vi "ReversedEngineering GetStateMachineCaseSelectorRefInfo.vi"(0 "Diagram":refnum<vi>, 1 "WhileLoop(False)":bool, 5 "error in (no error)":errorcluster) -> (12 "OutSideWhileLoopDiagram":refnum<vi>, 14 "StateWhileLoopDiagram":refnum<vi>, 15 "StateMachineCaseSelector":refnum<vi>, 16 "Found":bool, 19 "error out":errorcluster)   [LabVIEW 2016]
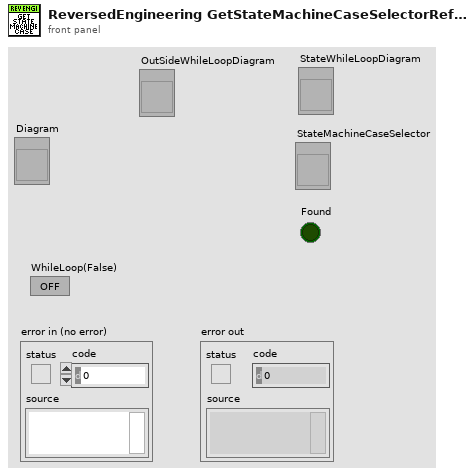
[diagram p1: front panel]
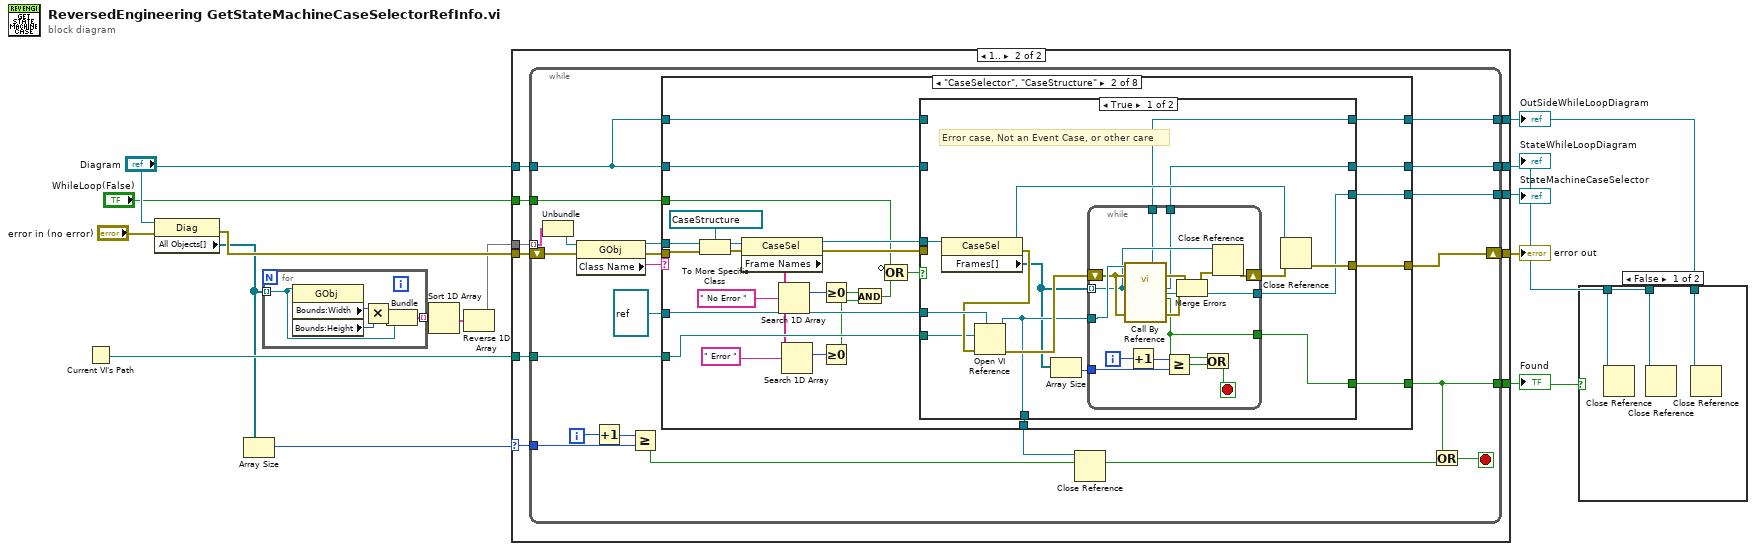
[diagram p0: block diagram]
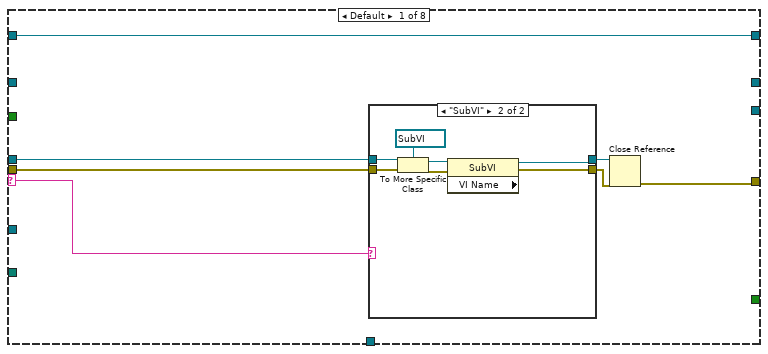
[diagram p3: hidden frame]
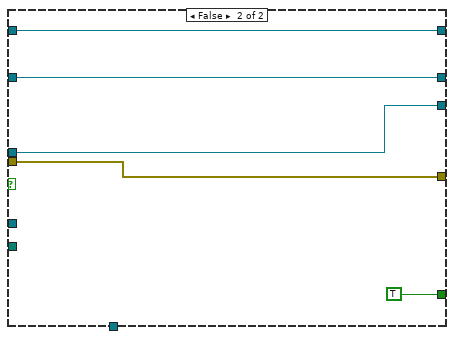
[diagram p5: hidden frame]
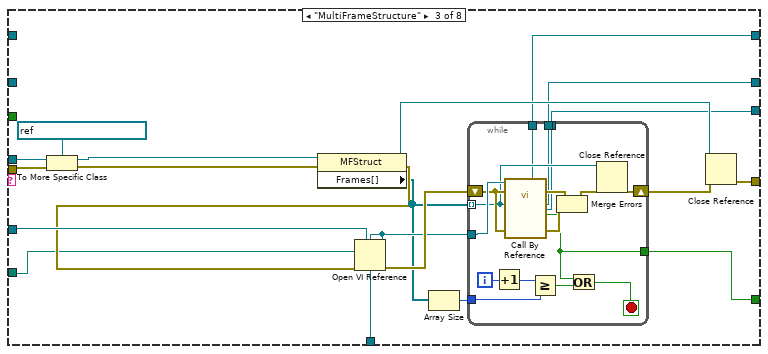
[diagram p6: hidden frame]
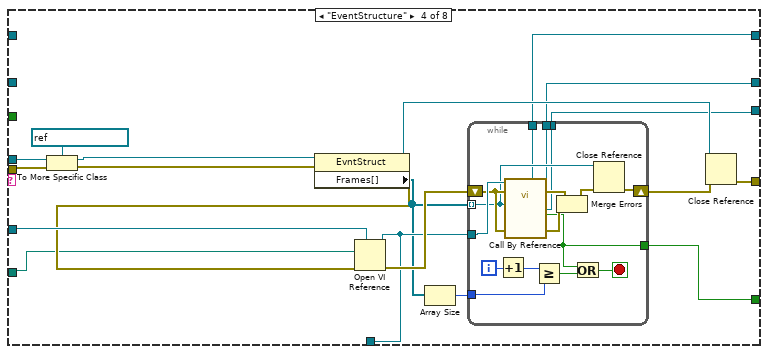
[diagram p7: hidden frame]
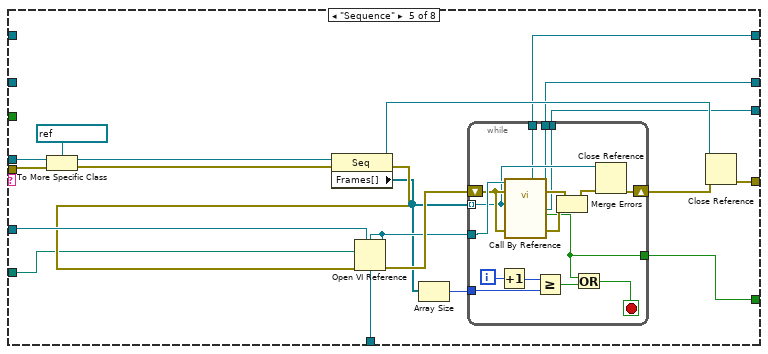
[diagram p8: hidden frame]
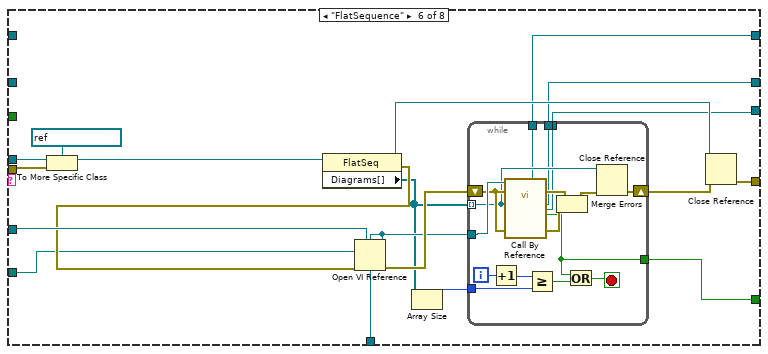
[diagram p9: hidden frame]
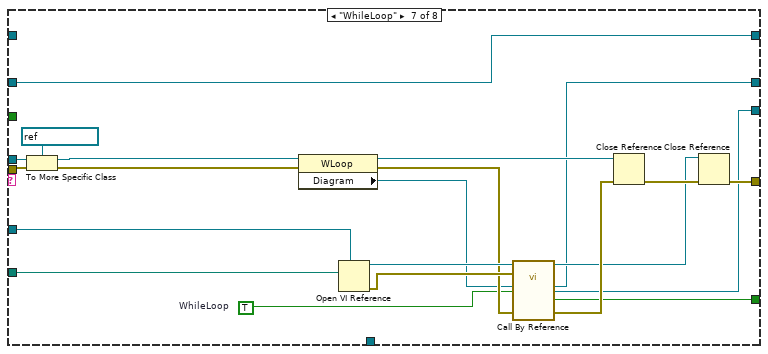
[diagram p10: hidden frame]
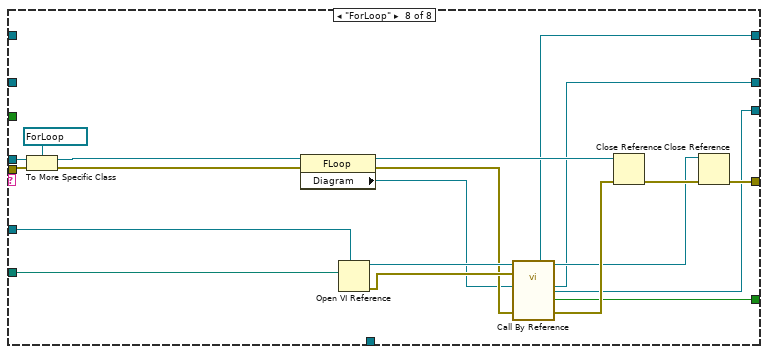
[diagram p11: hidden frame]
diagram:
  n1 = Current VI's Path() -> (path=w12:path)
  n2 = property class="Diag"(reference="Diagram", error in="error in (no error)") -> (error out=w14:errorcluster, "All Objects[]"=w2:refnum<vi>[])  [unwired: 1 out]
  n3 = Array Size(array=w2) -> (size(s)=w5:i32)
  n4 = for {
    tunnel: w2 -> [w16] mode=indexing
    tunnel: [w17] -> w4 mode=indexing
    n5 = property class="GObj"(reference=w16) -> ("Bounds:Width"=w20:u32, "Bounds:Height"=w19:u32)  [unwired: 1 in, 2 out]
    n6 = Multiply(x=w20, y=w19) -> (x*y=w18:u32)
    n7 = Bundle(w18, w16) -> (w17:cluster{u32, refnum<vi>})  [unwired: 1 out]
  }
  n8 = Sort 1D Array(array=w4) -> (sorted array=w3:cluster{u32, refnum<vi>}[])
  n9 = Reverse 1D Array(array=w3) -> (reversed array=w1:cluster{u32, refnum<vi>}[])
  n10 = case shown="1.." w5 {
    selector: w5 -> [_ w23]
    tunnel: w14 -> [w22 w33]
    tunnel: [w22 w32] -> w13
    tunnel: w12 -> [_ w31]
    tunnel: w1 -> [_ w30]
    tunnel: "Diagram" -> [w21 w29]
    tunnel: [_ w28] -> w10
    tunnel: [_ w27] -> w9
    tunnel: [_ w26] -> w8
    tunnel: [w21 w25] -> w7
    tunnel: "WhileLoop(False)" -> [_ w24]
    frame 0, Default {
    }
    frame 1.. {
      n11 = while {
        tunnel: w30 -> [w54] mode=indexing
        shift-right: [w49] -> w32
        shift-left: w33 -> [w51]
        tunnel: w31 -> [w47]
        tunnel: w23 -> [w43]
        tunnel: [w40] -> w27
        tunnel: [w39] -> w28
        tunnel: [w38] -> w25
        tunnel: [w37] -> w26
        tunnel: w29 -> [w36]
        tunnel: w24 -> [w35]
        i -> [w45]
        stop <- w41 stop-if-true
        n12 = Unbundle(w54) -> (w34:refnum<vi>)  [unwired: 1 out]
        n13 = property class="GObj"(reference=w34, error in=w51) -> (reference out=w52:refnum<vi>, error out=w50:errorcluster, "Class Name"=w53:string)
        n14 = Increment(x=w45) -> (x+1=w44:i32)
        n15 = Greater Or Equal?(x=w44, y=w43) -> (x >= y?=w42:bool)
        n16 = case shown="\"CaseSelector\", \"CaseStructure\"" w53 {
          selector: w53 -> [w60 _ _ _ _ _ _ _]
          tunnel: w52 -> [w58 w97 w152 w187 w222 w256 w293 w313]
          tunnel: w50 -> [w59 w96 w149 w184 w219 w255 w287 w307]
          tunnel: [w61 w95 w148 w183 w218 w254 w280 w300] -> w49
          tunnel: refnum<vi> refnum ("VI Refnum") -> [_ w94 w145 w180 w215 w252 w282 w302]
          tunnel: w47 -> [_ w93 w141 w176 w212 w246 w278 w298]
          tunnel: [_ w92 w140 w175 w210 w245 _ _] -> w46
          tunnel: [_ w88 w136 w171 w208 w243 w276 w296] -> w39
          tunnel: [_ w87 w137 w172 w209 w244 w277 w297] -> w40
          tunnel: w36 -> [_ w82 _ _ _ _ w274 _]
          tunnel: [_ w81 w135 w170 w205 w240 w275 w295] -> w37
          tunnel: w36 -> [w55 w75 _ _ _ _ _ _]
          tunnel: [w55 w74 w134 w169 w204 w239 w274 w294] -> w38
          tunnel: w35 -> [_ w71 _ _ _ _ _ _]
          frame Default {
            n17 = case shown="\"SubVI\"" w60 {
              tunnel: w59 -> [w63 w68]
              tunnel: w58 -> [w62 w69]
              tunnel: [w63 w66] -> w57
              tunnel: [w62 w65] -> w56
              frame "False", Default {
              }
              frame "SubVI" {
                n18 = To More Specific Class(target class=refnum<vi> refnum ("WhileLoop"), reference=w69, error in=w68) -> (specific class reference=w67:refnum<vi>, error out=w64:errorcluster)
                n19 = property class="SubVI" props=["VI Name"](reference=w67, error in=w64) -> (reference out=w65:refnum<vi>, error out=w66:errorcluster)  [unwired: 1 out]
              }
            }
            n20 = Close Reference(reference=w56, error in (no error)=w57) -> (error out=w61:errorcluster)
          }
          frame "CaseSelector", "CaseStructure" {
            n21 = To More Specific Class(target class=refnum<vi> refnum ("CaseSelector"), reference=w97, error in=w96) -> (specific class reference=w84:refnum<vi>, error out=w83:errorcluster)
            n22 = property class="CaseSel"(reference=w84, error in=w83) -> (reference out=w86:refnum<vi>, error out=w85:errorcluster, "Frame Names"=w80:string[])
            n23 = Search 1D Array(1D array=w80, element=" No Error ") -> (index of element=w89:i32)  [unwired: 1 in]
            n24 = Search 1D Array(1D array=w80, element=" Error ") -> (index of element=w77:i32)  [unwired: 1 in]
            n25 = Greater Or Equal To 0?(x=w89) -> (x >= 0?=w78:bool)
            n26 = Greater Or Equal To 0?(x=w77) -> (x >= 0?=w76:bool)
            n27 = And(x=w78, y=w76) -> (x .and. y?=w73:bool)
            n28 = Compound Arithmetic op=OR(invert w71, w73) -> (w72:bool)
            n29 = case shown="True" w72 {
              tunnel: [w112 w131] -> w95
              tunnel: w94 -> [w109 _]
              tunnel: w93 -> [w106 _]
              tunnel: [w105 _] -> w92
              tunnel: [w100 TRUE] -> w88
              tunnel: [w101 w132] -> w87
              tunnel: w86 -> [w104 w132]
              tunnel: w85 -> [_ w131]
              tunnel: w82 -> [_ w130]
              tunnel: [w99 w130] -> w81
              tunnel: w75 -> [_ w129]
              tunnel: [w98 w129] -> w74
              frame True {
                # "Error case, Not an Event Case, or other care"
                n30 = property class="CaseSel"(reference=w104) -> (reference out=w110:refnum<vi>, error out=w108:errorcluster, "Frames[]"=w103:refnum<vi>[])  [unwired: 1 in]
                n31 = Open VI Reference(type specifier VI Refnum (for type only)=w109, vi path=w106, error in (no error)=w108) -> (vi reference=w105:refnum<vi>, error out=w111:errorcluster)  [unwired: 3 out]
                n32 = Array Size(array=w103) -> (size(s)=w102:i32)
                n33 = while {
                  tunnel: w103 -> [w122] mode=indexing
                  shift-right: [w124] -> w107
                  shift-left: w111 -> [w126]
                  tunnel: w105 -> [w127]
                  tunnel: w102 -> [w119]
                  tunnel: [w116] -> w101
                  tunnel: [w115] -> w100
                  tunnel: [w114] -> w99
                  tunnel: [w113] -> w98
                  i -> [w120]
                  stop <- w118 stop-if-true
                  n34 = call-by-ref "?"(reference=w127, error in=w126, "Diagram"=w122, "error in (no error)"=w126) -> (error out=w128:errorcluster, "OutSideWhileLoopDiagram"=w113:refnum<vi>, "StateWhileLoopDiagram"=w114:refnum<vi>, "StateMachineCaseSelector"=w116:refnum<vi>, "Found"=w115:bool, 19:"error out"=w125:errorcluster)  [unwired: 13 in, 1 out]
                  n35 = Increment(x=w120) -> (x+1=w121:i32)
                  n36 = Greater Or Equal?(x=w121, y=w119) -> (x >= y?=w117:bool)
                  n37 = Merge Errors(w128, w125) -> (w123:errorcluster)
                  n38 = Or(x=w115, y=w117) -> (x .or. y?=w118:bool)
                  n39 = Close Reference(reference=w122, error in (no error)=w123) -> (error out=w124:errorcluster)
                }
                n40 = Close Reference(reference=w110, error in (no error)=w107) -> (error out=w112:errorcluster)
              }
              frame False {
              }
            }
          }
          frame "MultiFrameStructure" {
            n41 = To More Specific Class(target class=refnum<vi> refnum ("MultiFrameStructure"), reference=w152, error in=w149) -> (specific class reference=w151:refnum<vi>, error out=w150:errorcluster)
            n42 = property class="MFStruct"(reference=w151, error in=w150) -> (reference out=w146:refnum<vi>, error out=w144:errorcluster, "Frames[]"=w139:refnum<vi>[])
            n43 = Open VI Reference(type specifier VI Refnum (for type only)=w145, vi path=w141, error in (no error)=w144) -> (vi reference=w140:refnum<vi>, error out=w147:errorcluster)  [unwired: 3 out]
            n44 = Array Size(array=w139) -> (size(s)=w138:i32)
            n45 = while {
              tunnel: w139 -> [w164] mode=indexing
              shift-right: [w162] -> w143
              shift-left: w147 -> [w166]
              tunnel: w140 -> [w167]
              tunnel: w138 -> [w158]
              tunnel: [w156] -> w137
              tunnel: [w155] -> w136
              tunnel: [w154] -> w135
              tunnel: [w153] -> w134
              i -> [w159]
              stop <- w157 stop-if-true
              n46 = Increment(x=w159) -> (x+1=w161:i32)
              n47 = call-by-ref "?"(reference=w167, error in=w166, "Diagram"=w164, "error in (no error)"=w166) -> (error out=w168:errorcluster, "OutSideWhileLoopDiagram"=w153:refnum<vi>, "StateWhileLoopDiagram"=w154:refnum<vi>, "StateMachineCaseSelector"=w156:refnum<vi>, "Found"=w155:bool, 19:"error out"=w165:errorcluster)  [unwired: 13 in, 1 out]
              n48 = Greater Or Equal?(x=w161, y=w158) -> (x >= y?=w160:bool)
              n49 = Merge Errors(w168, w165) -> (w163:errorcluster)
              n50 = Or(x=w155, y=w160) -> (x .or. y?=w157:bool)
              n51 = Close Reference(reference=w164, error in (no error)=w163) -> (error out=w162:errorcluster)
            }
            n52 = Close Reference(reference=w146, error in (no error)=w143) -> (error out=w148:errorcluster)
          }
          frame "EventStructure" {
            n53 = To More Specific Class(target class=refnum<vi> refnum ("EventStructure"), reference=w187, error in=w184) -> (specific class reference=w186:refnum<vi>, error out=w185:errorcluster)
            n54 = property class="EvntStruct"(reference=w186, error in=w185) -> (reference out=w181:refnum<vi>, error out=w179:errorcluster, "Frames[]"=w174:refnum<vi>[])
            n55 = Open VI Reference(type specifier VI Refnum (for type only)=w180, vi path=w176, error in (no error)=w179) -> (vi reference=w175:refnum<vi>, error out=w182:errorcluster)  [unwired: 3 out]
            n56 = Array Size(array=w174) -> (size(s)=w173:i32)
            n57 = while {
              tunnel: w174 -> [w197] mode=indexing
              shift-right: [w198] -> w178
              shift-left: w182 -> [w201]
              tunnel: w175 -> [w202]
              tunnel: w173 -> [w193]
              tunnel: [w192] -> w172
              tunnel: [w191] -> w171
              tunnel: [w189] -> w170
              tunnel: [w188] -> w169
              i -> [w194]
              stop <- w190 stop-if-true
              n58 = Increment(x=w194) -> (x+1=w196:i32)
              n59 = call-by-ref "?"(reference=w202, error in=w201, "Diagram"=w197, "error in (no error)"=w201) -> (error out=w203:errorcluster, "OutSideWhileLoopDiagram"=w188:refnum<vi>, "StateWhileLoopDiagram"=w189:refnum<vi>, "StateMachineCaseSelector"=w192:refnum<vi>, "Found"=w191:bool, 19:"error out"=w200:errorcluster)  [unwired: 13 in, 1 out]
              n60 = Greater Or Equal?(x=w196, y=w193) -> (x >= y?=w195:bool)
              n61 = Merge Errors(w203, w200) -> (w199:errorcluster)
              n62 = Or(x=w191, y=w195) -> (x .or. y?=w190:bool)
              n63 = Close Reference(reference=w197, error in (no error)=w199) -> (error out=w198:errorcluster)
            }
            n64 = Close Reference(reference=w181, error in (no error)=w178) -> (error out=w183:errorcluster)
          }
          frame "Sequence" {
            n65 = To More Specific Class(target class=refnum<vi> refnum ("Sequence"), reference=w222, error in=w219) -> (specific class reference=w221:refnum<vi>, error out=w220:errorcluster)
            n66 = property class="Seq"(reference=w221, error in=w220) -> (reference out=w216:refnum<vi>, error out=w214:errorcluster, "Frames[]"=w207:refnum<vi>[])
            n67 = Open VI Reference(type specifier VI Refnum (for type only)=w215, vi path=w212, error in (no error)=w214) -> (vi reference=w210:refnum<vi>, error out=w217:errorcluster)  [unwired: 3 out]
            n68 = Array Size(array=w207) -> (size(s)=w206:i32)
            n69 = while {
              tunnel: w207 -> [w232] mode=indexing
              shift-right: [w234] -> w211
              shift-left: w217 -> [w236]
              tunnel: w210 -> [w237]
              tunnel: [w227] -> w209
              tunnel: [w226] -> w208
              tunnel: w206 -> [w225]
              tunnel: [w224] -> w205
              tunnel: [w223] -> w204
              i -> [w229]
              stop <- w228 stop-if-true
              n70 = Increment(x=w229) -> (x+1=w231:i32)
              n71 = call-by-ref "?"(reference=w237, error in=w236, "Diagram"=w232, "error in (no error)"=w236) -> (error out=w238:errorcluster, "OutSideWhileLoopDiagram"=w223:refnum<vi>, "StateWhileLoopDiagram"=w224:refnum<vi>, "StateMachineCaseSelector"=w227:refnum<vi>, "Found"=w226:bool, 19:"error out"=w235:errorcluster)  [unwired: 13 in, 1 out]
              n72 = Greater Or Equal?(x=w231, y=w225) -> (x >= y?=w230:bool)
              n73 = Merge Errors(w238, w235) -> (w233:errorcluster)
              n74 = Or(x=w226, y=w230) -> (x .or. y?=w228:bool)
              n75 = Close Reference(reference=w232, error in (no error)=w233) -> (error out=w234:errorcluster)
            }
            n76 = Close Reference(reference=w216, error in (no error)=w211) -> (error out=w218:errorcluster)
          }
          frame "FlatSequence" {
            n77 = To More Specific Class(target class=refnum<vi> refnum ("FlatSequence"), reference=w256, error in=w255) -> (specific class reference=w249:refnum<vi>)  [unwired: 1 out]
            n78 = property class="FlatSeq"(reference=w249) -> (reference out=w247:refnum<vi>, error out=w248:errorcluster, "Diagrams[]"=w242:refnum<vi>[])  [unwired: 1 in]
            n79 = Open VI Reference(type specifier VI Refnum (for type only)=w252, vi path=w246, error in (no error)=w248) -> (vi reference=w245:refnum<vi>, error out=w253:errorcluster)  [unwired: 3 out]
            n80 = Array Size(array=w242) -> (size(s)=w241:i32)
            n81 = while {
              tunnel: w242 -> [w266] mode=indexing
              shift-right: [w268] -> w251
              shift-left: w253 -> [w270]
              tunnel: w245 -> [w271]
              tunnel: [w261] -> w244
              tunnel: [w260] -> w243
              tunnel: w241 -> [w259]
              tunnel: [w258] -> w240
              tunnel: [w257] -> w239
              i -> [w263]
              stop <- w262 stop-if-true
              n82 = Increment(x=w263) -> (x+1=w265:i32)
              n83 = call-by-ref "?"(reference=w271, error in=w270, "Diagram"=w266, "error in (no error)"=w270) -> (error out=w272:errorcluster, "OutSideWhileLoopDiagram"=w257:refnum<vi>, "StateWhileLoopDiagram"=w258:refnum<vi>, "StateMachineCaseSelector"=w261:refnum<vi>, "Found"=w260:bool, 19:"error out"=w269:errorcluster)  [unwired: 13 in, 1 out]
              n84 = Greater Or Equal?(x=w265, y=w259) -> (x >= y?=w264:bool)
              n85 = Merge Errors(w272, w269) -> (w267:errorcluster)
              n86 = Or(x=w260, y=w264) -> (x .or. y?=w262:bool)
              n87 = Close Reference(reference=w266, error in (no error)=w267) -> (error out=w268:errorcluster)
            }
            n88 = Close Reference(reference=w247, error in (no error)=w251) -> (error out=w254:errorcluster)
          }
          frame "WhileLoop" {
            w273 = TRUE  # WhileLoop
            n89 = To More Specific Class(target class=refnum<vi> refnum ("WhileLoop"), reference=w293, error in=w287) -> (specific class reference=w292:refnum<vi>, error out=w288:errorcluster)
            n90 = property class="WLoop"(reference=w292, error in=w288) -> (reference out=w290:refnum<vi>, error out=w284:errorcluster, "Diagram"=w283:refnum<vi>)
            n91 = Open VI Reference(type specifier VI Refnum (for type only)=w282, vi path=w278) -> (vi reference=w286:refnum<vi>, error out=w289:errorcluster)  [unwired: 1 in, 3 out]
            n92 = call-by-ref "?"(reference=w286, error in=w289, "Diagram"=w283, "WhileLoop(False)"=w273, "error in (no error)"=w284) -> (reference out=w279:refnum<vi>, "StateWhileLoopDiagram"=w275:refnum<vi>, "StateMachineCaseSelector"=w277:refnum<vi>, "Found"=w276:bool, "error out"=w285:errorcluster)  [unwired: 12 in, 2 out]
            n93 = Close Reference(reference=w290, error in (no error)=w285) -> (error out=w281:errorcluster)
            n94 = Close Reference(reference=w279, error in (no error)=w281) -> (error out=w280:errorcluster)
          }
          frame "ForLoop" {
            n95 = To More Specific Class(target class=refnum<vi> refnum ("WhileLoop"), reference=w313, error in=w307) -> (specific class reference=w312:refnum<vi>, error out=w308:errorcluster)
            n96 = property class="FLoop"(reference=w312, error in=w308) -> (reference out=w310:refnum<vi>, error out=w304:errorcluster, "Diagram"=w303:refnum<vi>)
            n97 = Open VI Reference(type specifier VI Refnum (for type only)=w302, vi path=w298) -> (vi reference=w306:refnum<vi>, error out=w309:errorcluster)  [unwired: 1 in, 3 out]
            n98 = call-by-ref "?"(reference=w306, error in=w309, "Diagram"=w303, "error in (no error)"=w304) -> (reference out=w299:refnum<vi>, "OutSideWhileLoopDiagram"=w294:refnum<vi>, "StateWhileLoopDiagram"=w295:refnum<vi>, "StateMachineCaseSelector"=w297:refnum<vi>, "Found"=w296:bool, "error out"=w305:errorcluster)  [unwired: 13 in, 1 out]
            n99 = Close Reference(reference=w310, error in (no error)=w305) -> (error out=w301:errorcluster)
            n100 = Close Reference(reference=w299, error in (no error)=w301) -> (error out=w300:errorcluster)
          }
        }
        n101 = Close Reference(reference=w46) -> ()  [unwired: 1 in, 1 out]
        n102 = Or(x=w39, y=w42) -> (x .or. y?=w41:bool)
      }
    }
  }
  "error out" <- w13
  "StateMachineCaseSelector" <- w9
  "Found" <- w10
  "StateWhileLoopDiagram" <- w8
  "OutSideWhileLoopDiagram" <- w7
  n103 = case shown="False" w10 {
    tunnel: w9 -> [w316 _]
    tunnel: w8 -> [w315 _]
    tunnel: w7 -> [w314 _]
    frame False {
      n104 = Close Reference(reference=w316) -> ()  [unwired: 1 in, 1 out]
      n105 = Close Reference(reference=w315) -> ()  [unwired: 1 in, 1 out]
      n106 = Close Reference(reference=w314) -> ()  [unwired: 1 in, 1 out]
    }
    frame True {
    }
  }
